vi "Directory of Top Level VI.vi"(0 "error in (no error)":errorcluster) -> (1 "directory of top VI":path, 2 "error out":errorcluster)   [LabVIEW 2014]
doc: "This VI will get the directory in which the top level VI of the program is contained. If VI is in a library (.llb) file the directory in which the library file exists is returned"
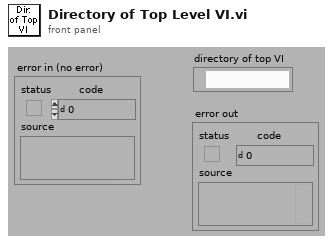
[diagram p1: front panel]
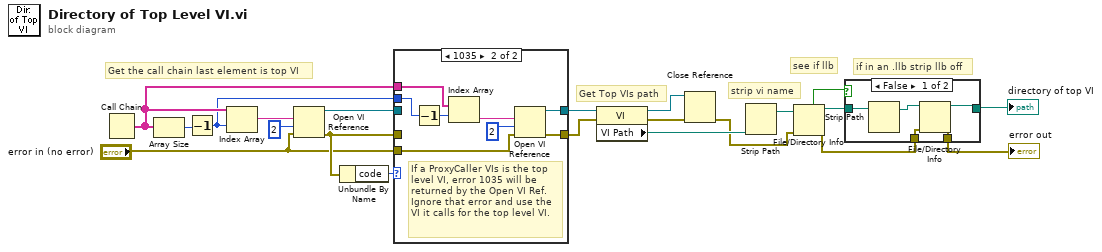
[diagram p0: block diagram]
diagram:
  # "if in an .llb strip llb off"
  # "see if llb"
  # "strip vi name"
  # "Get Top VIs path"
  # "Get the call chain last element is top VI"
  n1 = Call Chain() -> (call chain=w8:string[])
  n2 = Array Size(array=w8) -> (size(s)=w15:i32)
  n3 = Decrement(x=w15) -> (x-1=w7:i32)
  n4 = Index Array(array=w8, index=w7) -> (element=w16:string)
  n5 = Open VI Reference(vi path=w16, options=2, error in (no error)="error in (no error)") -> (vi reference=w10:refnum<vi>, error out=w9:errorcluster)  [unwired: 3 in]
  n6 = Unbundle By Name(w9) -> ("code"=w11:i32)
  n7 = case shown="1035" w11 {
    tunnel: [w23 w26] -> w6
    tunnel: w10 -> [w23 _]
    tunnel: [w22 w27] -> w5
    tunnel: w9 -> [w22 _]
    tunnel: w8 -> [_ w30]
    tunnel: w7 -> [_ w29]
    tunnel: "error in (no error)" -> [_ w24]
    frame 0, Default {
    }
    frame 1035 {
      # "If a ProxyCaller VIs is the top\nlevel VI, error 1035 will be\nreturned by the Open VI Ref.\nIgnore that error and use the\nVI it calls for the top level VI."
      n8 = Decrement(x=w29) -> (x-1=w31:i32)
      n9 = Index Array(array=w30, index=w31) -> (element=w28:string)
      n10 = Open VI Reference(vi path=w28, options=2, error in (no error)=w24) -> (vi reference=w26:refnum<vi>, error out=w27:errorcluster)  [unwired: 3 in]
    }
  }
  n11 = property class="VI"(reference=w6, error in=w5) -> (reference out=w1:refnum<vi>, error out=w3:errorcluster, "VI Path"=w20:path)
  n12 = Close Reference(reference=w1, error in (no error)=w3) -> (error out=w2:errorcluster)
  n13 = Strip Path(path=w20) -> (stripped path=w17:path)  [unwired: 1 out]
  n14 = File/Directory Info(path=w17, error in=w2) -> (path out=w19:path, directory=w18:bool, error out=w14:errorcluster)  [unwired: 4 out]
  n15 = case shown="False" w18 {
    tunnel: w19 -> [w36 w38]
    tunnel: [w32 w38] -> w21
    tunnel: w14 -> [w34 w37]
    tunnel: [w33 w37] -> w13
    frame False {
      n16 = Strip Path(path=w36) -> (stripped path=w35:path)  [unwired: 1 out]
      n17 = File/Directory Info(path=w35, error in=w34) -> (path out=w32:path, error out=w33:errorcluster)  [unwired: 5 out]
    }
    frame True {
    }
  }
  "error out" <- w13
  "directory of top VI" <- w21
